vi "llh2XYZ.vi"(9 "llh":dbl[](array[numeric])=[0.0, 0.0, 0.0]) -> (2 "DCM(ecef2lcc)":dbl[][](array[numeric]), 3 "ecef":dbl[](array[numeric]) format="%#_19f")   [LabVIEW 2012]
panel:
  out "cos(phi)":dbl
  out "sin(phi)":dbl
  out "sin(lam)":dbl
  out "cos(lam)":dbl
  out "hgt":dbl
  out "b^2/a^2":dbl
  out "N":dbl format="%#_19f"
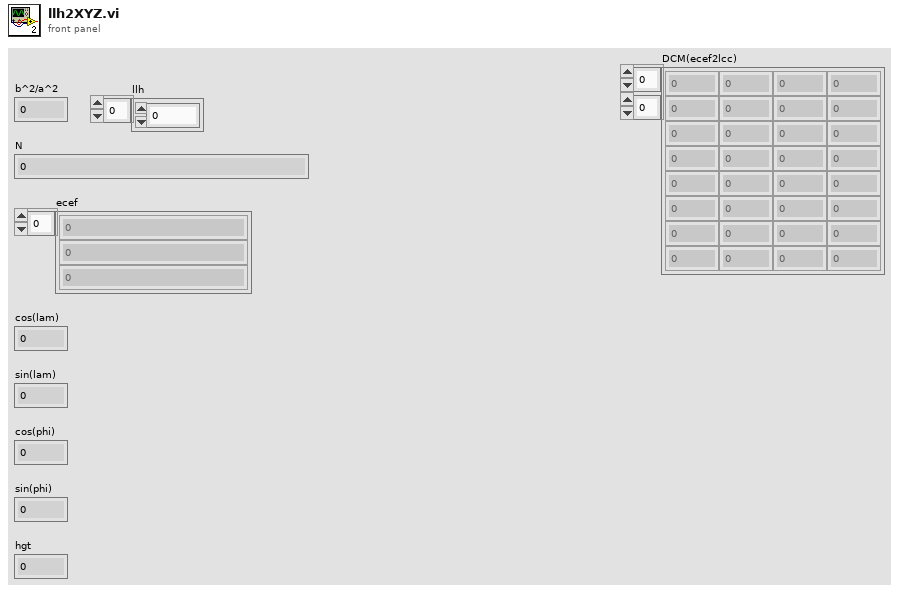
[diagram p1: front panel]
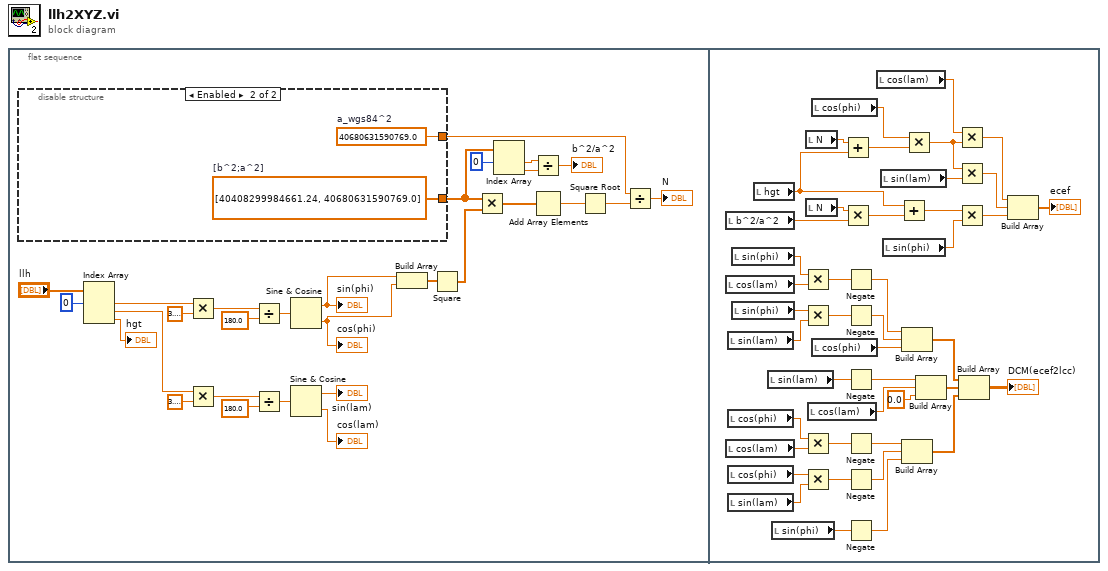
[diagram p0: block diagram]
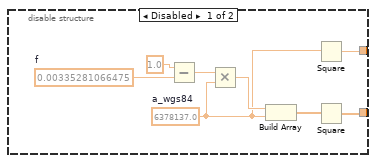
[diagram p2: hidden frame]
diagram:
  n1 = flat-sequence {
    frame #0 {
      n2 = disable-structure shown="Enabled" {
        disable-tunnel: [w32 w39] -> w19
        disable-tunnel: [w30 w38] -> w16
        frame Disabled {
          w37 = 0.00335281066475  # f
          w31 = 6378137.0  # a_wgs84
          n3 = Subtract(x=1.0, y=w37) -> (x-y=w35:dbl)
          n4 = Multiply(x=w35, y=w31) -> (x*y=w34:dbl)
          n5 = Build Array(w34, w31) -> (w33:dbl[])
          n6 = Square(x=w31) -> (x^2=w30:dbl)
          n7 = Square(x=w33) -> (x^2=w32:dbl[])
        }
        frame Enabled {
          w38 = 40680631590769.0  # a_wgs84^2
          w39 = dbl[] [40408299984661.24, 40680631590769.0]  # [b^2;a^2]
        }
      }
      n8 = Index Array(array="llh", index #1=0 ("index")) -> (element #1=w3:dbl, element #2=w2:dbl, element #3=→"hgt":dbl)  [unwired: 2 in]
      n9 = Multiply(x=w3, y=3.141592653589793) -> (x*y=w7:dbl)
      n10 = Multiply(x=w2, y=3.141592653589793) -> (x*y=w26:dbl)
      n11 = Divide(x=w7, y=180.0) -> (x/y=w9:dbl)
      n12 = Divide(x=w26, y=180.0) -> (x/y=w24:dbl)
      n13 = Sine & Cosine(0:w9) -> (1:w10:dbl, 2:w11:dbl)
      "sin(phi)" <- w10
      "cos(phi)" <- w11
      n14 = Sine & Cosine(0:w24) -> (1:→"sin(lam)":dbl, 2:→"cos(lam)":dbl)
      n15 = Build Array(w10, w11) -> (w12:dbl[])
      n16 = Square(x=w12) -> (x^2=w13:dbl[])
      n17 = Multiply(x=w19, y=w13) -> (x*y=w18:dbl[])
      n18 = Index Array(array=w19, index #1=0 ("index")) -> (element #1=w21:dbl, element #2=w22:dbl)  [unwired: 1 in]
      n19 = Divide(x=w21, y=w22) -> (x/y=→"b^2/a^2":dbl)
      n20 = Add Array Elements(numeric array=w18) -> (sum=w14:dbl)
      n21 = Square Root(x=w14) -> (sqrt(x)=w17:dbl)
      n22 = Divide(x=w16, y=w17) -> (x/y=→"N":dbl)
    }
    frame #1 {
      n23 = local read "b^2/a^2"() -> (w71:dbl)
      n24 = local read "cos(lam)"() -> (w65:dbl)
      n25 = local read "cos(lam)"() -> (w47:dbl)
      n26 = local read "sin(lam)"() -> (w62:dbl)
      n27 = local read "cos(phi)"() -> (w46:dbl)
      n28 = local read "cos(phi)"() -> (w51:dbl)
      n29 = local read "sin(lam)"() -> (w50:dbl)
      n30 = local read "sin(phi)"() -> (w66:dbl)
      n31 = local read "sin(phi)"() -> (w61:dbl)
      n32 = local read "hgt"() -> (w74:dbl)
      n33 = local read "sin(lam)"() -> (w57:dbl)
      n34 = local read "sin(phi)"() -> (w45:dbl)
      n35 = Multiply(x=w66, y=w65) -> (x*y=w64:dbl)
      n36 = Multiply(x=w61, y=w62) -> (x*y=w63:dbl)
      n37 = Multiply(x=w46, y=w47) -> (x*y=w48:dbl)
      n38 = Multiply(x=w51, y=w50) -> (x*y=w49:dbl)
      n39 = local read "N"() -> (w73:dbl)
      n40 = local read "N"() -> (w72:dbl)
      n41 = local read "cos(lam)"() -> (w55:dbl)
      n42 = local read "cos(phi)"() -> (w69:dbl)
      n43 = local read "cos(phi)"() -> (w58:dbl)
      n44 = Add(x=w73, y=w74) -> (x+y=w82:dbl)
      n45 = Multiply(x=w72, y=w71) -> (x*y=w78:dbl)
      n46 = Negate(x=w64) -> (-x=w60:dbl)
      n47 = Negate(x=w63) -> (-x=w59:dbl)
      n48 = Negate(x=w57) -> (-x=w56:dbl)
      n49 = Negate(x=w48) -> (-x=w52:dbl)
      n50 = Negate(x=w49) -> (-x=w53:dbl)
      n51 = Negate(x=w45) -> (-x=w44:dbl)
      n52 = local read "cos(lam)"() -> (w68:dbl)
      n53 = local read "sin(lam)"() -> (w67:dbl)
      n54 = local read "sin(phi)"() -> (w70:dbl)
      n55 = Add(x=w74, y=w78) -> (x+y=w77:dbl)
      n56 = Build Array(w60, w59, w58) -> (w43:dbl[])
      n57 = Build Array(w52, w53, w44) -> (w41:dbl[])
      n58 = Multiply(x=w69, y=w82) -> (x*y=w81:dbl)
      n59 = Build Array(w56, w55, 0.0 ("element")) -> (w42:dbl[])
      n60 = Multiply(x=w68, y=w81) -> (x*y=w80:dbl)
      n61 = Multiply(x=w81, y=w67) -> (x*y=w79:dbl)
      n62 = Multiply(x=w77, y=w70) -> (x*y=w76:dbl)
      n63 = Build Array(w43, w42, w41) -> (→"DCM(ecef2lcc)":dbl[][])
      n64 = Build Array(w80, w79, w76) -> (→"ecef":dbl[])
    }
  }
